vi "Save BackUp.vi"(0 "Refnum in":refnum<visa-resource-name>, 5 "Mode":T1, 7 "file path (dialog if empty)":path, 11 "error in (no error)":errorcluster, 12 "Enable":bool) -> (4 "Refnum Out":refnum<visa-resource-name>, 6 "ModeOut":T1, 15 "error out":errorcluster)   [LabVIEW 2020]
uses:
  <vilib>/Utility/file.llb/Write Delimited Spreadsheet (string).vi
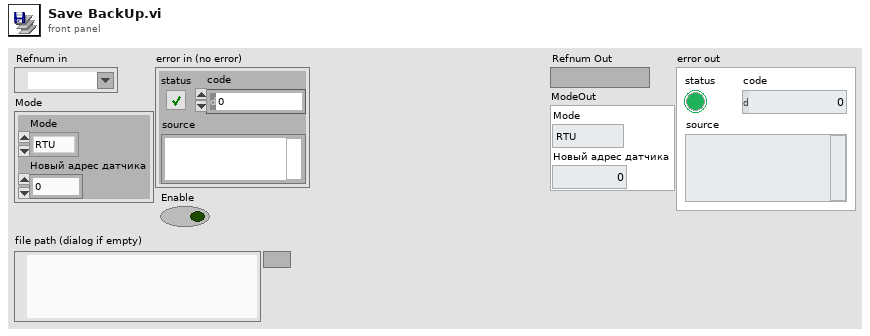
[diagram p1: front panel]
types:
  T1 = cluster{"Mode":enum16{"RTU", "ASCII"}, "Новый адрес датчика":u16}
  T2 = cluster{"Name":string, "Address":u16, "Type":u16, "Value":sgl}[]
  T3 = cluster{"Name":string, "Address":u16, "Type":u16, "Value":sgl}
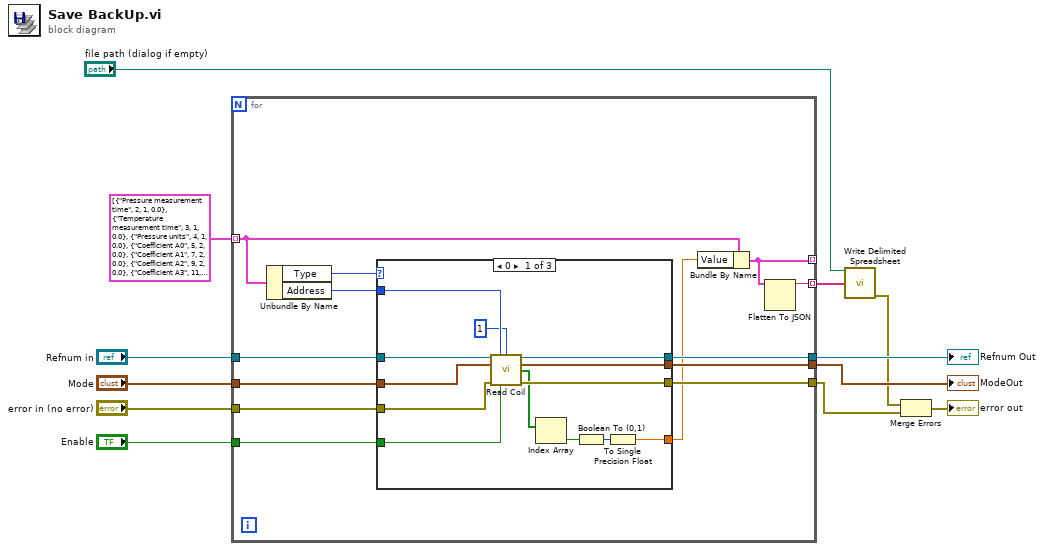
[diagram p0: block diagram]
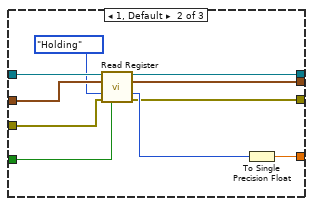
[diagram p2: hidden frame]
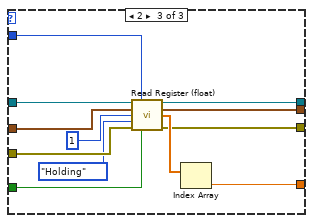
[diagram p3: hidden frame]
diagram:
  n1 = for {
    tunnel: T2 [{"Name"="Pressure measurement time", "Address"=2, "Type"=1, "Value"=0.0}, {"Name"="Temperature measurement time", "Address"=3, "Type"=1, "Value"=0.0}, {"Name"="Pressure units", "Address"=4, "Type"=1, "Value"=0.0}, {"Name"="Coefficient A0", "Address"=5, "Type"=2, "Value"=0.0}, {"Name"="Coefficient A1", "Address"=7, "Type"=2, "Value"=0.0}, {"Name"="Coefficient A2", "Address"=9, "Type"=2, "Value"=0.0}, {"Name"="Coefficient A3", "Address"=11, "Type"=2, "Value"=0.0}, {"Name"="Coefficient A4", "Address"=13, "Type"=2, "Value"=0.0}, {"Name"="Coefficient A5", "Address"=15, "Type"=2, "Value"=0.0}, {"Name"="Coefficient A6", "Address"=17, "Type"=2, "Value"=0.0}, {"Name"="Coefficient A7", "Address"=19, "Type"=2, "Value"=0.0}, {"Name"="Coefficient A8", "Address"=21, "Type"=2, "Value"=0.0}, {"Name"="Coefficient A9", "Address"=23, "Type"=2, "Value"=0.0}, {"Name"="Coefficient A10", "Address"=25, "Type"=2, "Value"=0.0}, {"Name"="Coefficient A11", "Address"=27, "Type"=2, "Value"=0.0}, {"Name"="Coefficient A12", "Address"=29, "Type"=2, "Value"=0.0}, {"Name"="Coefficient A13", "Address"=31, "Type"=2, "Value"=0.0}, {"Name"="Coefficient A14", "Address"=33, "Type"=2, "Value"=0.0}, {"Name"="Coefficient A15", "Address"=35, "Type"=2, "Value"=0.0}, {"Name"="Coefficient Ft0", "Address"=37, "Type"=2, "Value"=0.0}, {"Name"="Coefficient Fp0", "Address"=39, "Type"=2, "Value"=0.0}, {"Name"="Coefficient T0", "Address"=41, "Type"=2, "Value"=0.0}, {"Name"="Coefficient C1", "Address"=43, "Type"=2, "Value"=0.0}, {"Name"="Coefficient C2", "Address"=44, "Type"=2, "Value"=0.0}, {"Name"="Coefficient C3", "Address"=47, "Type"=2, "Value"=0.0}, {"Name"="Coefficient C4", "Address"=49, "Type"=2, "Value"=0.0}, {"Name"="Coefficient C5", "Address"=51, "Type"=2, "Value"=0.0}, {"Name"="Coefficient F0", "Address"=53, "Type"=2, "Value"=0.0}, {"Name"="Modbus Address", "Address"=55, "Type"=1, "Value"=0.0}, {"Name"="Baud rate", "Address"=56, "Type"=1, "Value"=0.0}, {"Name"="Auto send period", "Address"=57, "Type"=1, "Value"=0.0}, {"Name"="p_atm ", "Address"=62, "Type"=2, "Value"=0.0}, {"Name"="Pressure channel connection", "Address"=1, "Type"=0, "Value"=0.0}, {"Name"="Temperature channel connection", "Address"=2, "Type"=0, "Value"=0.0}, {"Name"="Continuous data output mode ", "Address"=5, "Type"=0, "Value"=0.0}, {"Name"="Energysave mode", "Address"=6, "Type"=0, "Value"=0.0}] ("Array") -> [w16] mode=indexing
    tunnel: "Refnum in" -> [w23]
    tunnel: "Mode" -> [w22]
    tunnel: "error in (no error)" -> [w21]
    tunnel: "Enable" -> [w20]
    tunnel: [w19] -> w7
    tunnel: [w18] -> w6
    tunnel: [w17] -> w3
    tunnel: [w14] -> _ mode=indexing
    tunnel: [w13] -> w5 mode=indexing
    n2 = Unbundle By Name(w16) -> ("Type"=w25:u16, "Address"=w24:u16)
    n3 = case shown="0" w25 {
      tunnel: w24 -> [w34 _ w60]
      tunnel: w23 -> [w38 w48 w59]
      tunnel: w22 -> [w37 w47 w58]
      tunnel: w21 -> [w32 w43 w57]
      tunnel: w20 -> [w26 w42 w56]
      tunnel: [w36 w46 w53] -> w19
      tunnel: [w35 w45 w52] -> w18
      tunnel: [w31 w39 w51] -> w17
      tunnel: [w27 w41 w50] -> w15
      frame 0 {
        n4 = call "Read Coil.vi"("Refnum in"=w38, "startReg"=w34, "Quantity"=u16 1, "Mode"=w37, "error in (no error)"=w32, "Enable"=w26) -> ("Refnum Out"=w36:refnum<visa-resource-name>, "ModeOut"=w35:T1, "Coils"=w30:bool[], "error out"=w31:errorcluster)  [unwired: 6 in]
        n5 = Index Array(array=w30) -> (element=w29:bool)  [unwired: 1 in]
        n6 = Boolean To (0,1)(Boolean=w29) -> (0, 1=w28:i16)
        n7 = To Single Precision Float(number=w28) -> (single precision float=w27:sgl)
      }
      frame 1, Default {
        n8 = call "Read Register.vi"("Refnum in"=w48, "Mode"=w47, "Register type"=enum16{"Input", "Holding"}."Holding", "error in (no error)"=w43, "Enable"=w42) -> ("Refnum Out"=w46:refnum<visa-resource-name>, "ModeOut"=w45:T1, "Numeric"=w40:u16, "error out"=w39:errorcluster)  [unwired: 6 in, 1 out]
        n9 = To Single Precision Float(number=w40) -> (single precision float=w41:sgl)
      }
      frame 2 {
        n10 = call "Read Register (float).vi"("Refnum in"=w59, "startReg"=w60, "Mode"=w58, "WordCount"=u16 1, "Register type"=enum16{"Input", "Holding"}."Holding", "error in (no error)"=w57, "Enable"=w56) -> ("Refnum Out"=w53:refnum<visa-resource-name>, "ModeOut"=w52:T1, "Data"=w54:sgl[], "error out"=w51:errorcluster)  [unwired: 4 in, 1 out]
        n11 = Index Array(array=w54) -> (element=w50:sgl)  [unwired: 1 in]
      }
    }
    n12 = Bundle By Name(cluster=w16, "Value"=w15) -> (w14:T3)
    n13 = Flatten To JSON(anything=w14) -> (JSON string=w13:string)  [unwired: 2 in, 1 out]
  }
  "Refnum Out" <- w7
  "ModeOut" <- w6
  n14 = call-poly <vilib>:"Write Delimited Spreadsheet.vi"("file path (dialog if empty)"="file path (dialog if empty)", "1D data"=w5) -> ("error out"=w2:errorcluster)  [unwired: 12 in, 1 out]
  n15 = Merge Errors(w2, w3) -> (→"error out":errorcluster)
